vi "REAS BARCODE STRING.vi"(0 "error in (no error)":errorcluster, 8 "Input":string, 9 "Enum":enum16{"Read", "Write"}(ring)) -> (3 "error out":errorcluster, 11 "Input 2":string)   [LabVIEW 2017]
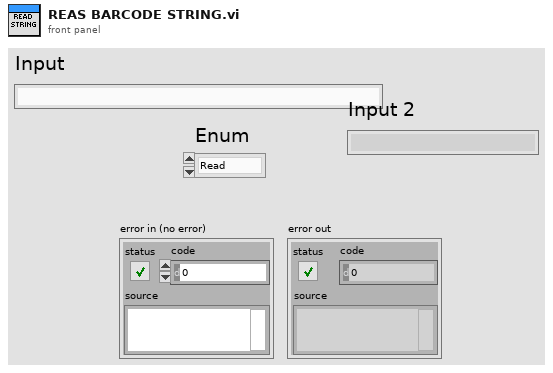
[diagram p1: front panel]
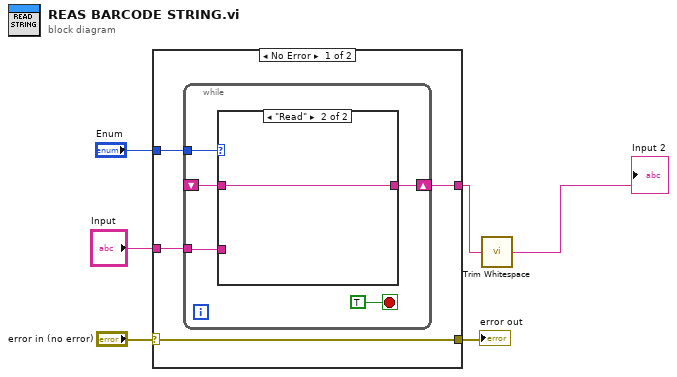
[diagram p0: block diagram]
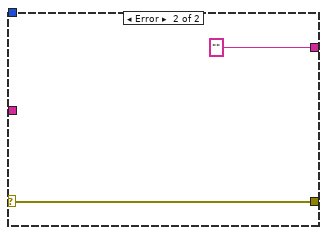
[diagram p3: hidden frame]
diagram:
  n1 = case shown="No Error" "error in (no error)" {
    selector: "error in (no error)" -> [w7 w18]
    tunnel: "Enum" -> [w10 _]
    tunnel: "Input" -> [w9 _]
    tunnel: [w8 ""] -> w1
    tunnel: [w7 w18] -> w4
    frame No Error {
      n2 = while {
        tunnel: w10 -> [w15]
        shift-right: [w13] -> w8
        shift-left: _ -> [w12]
        tunnel: w9 -> [w14]
        stop <- TRUE stop-if-true
        n3 = case shown="\"Read\"" w15 {
          tunnel: [w16 w17] -> w13
          tunnel: w14 -> [w16 _]
          tunnel: w12 -> [_ w17]
          frame "Write", Default {
          }
          frame "Read" {
          }
        }
      }
    }
    frame Error {
    }
  }
  "error out" <- w4
  n4 = call <vilib>:"Trim Whitespace.vi"("string"=w1) -> ("trimmed string"=→"Input 2":string)  [unwired: 1 in]
